vi "MixAndDownsample_5772.vi"(9 "Sine in":fxp<+/-,16,0>[](array[numeric])=[0.0, 0.0, 0.0, 0.0], 10 "Cosine in":fxp<+/-,16,0>[](array[numeric])=[0.0, 0.0, 0.0, 0.0], 11 "Signal Input":i16[](array[numeric])=[0, 0, 0, 0]) -> (0 "data valid":bool, 1 "Q out":fxp<+/-,16,14>, 2 "I out":fxp<+/-,16,14>)   [LabVIEW 2013]
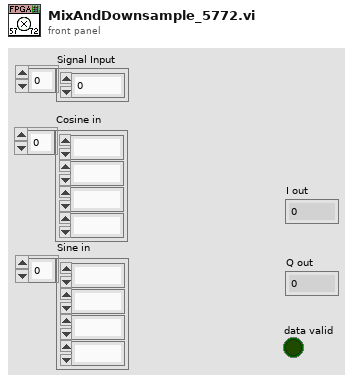
[diagram p1: front panel]
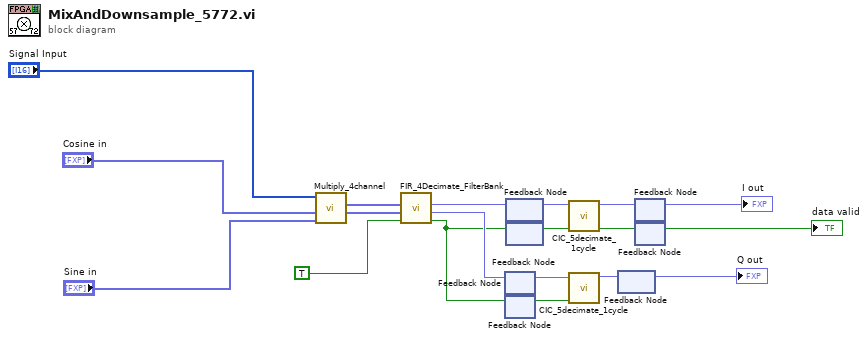
[diagram p0: block diagram]
diagram:
  n1 = call "Multiply_4channel.vi"("DDS Sine"="Sine in", "DDS Cosine"="Cosine in", "Signal Input"="Signal Input") -> ("Q output"=w15:fxp<+/-,16,14>[], "I output"=w16:fxp<+/-,16,14>[])  [unwired: 7 in]
  n2 = call "FIR_4Decimate_FilterBank.vi"("data valid in"=TRUE ("valid in"), "Q in"=w15, "I in"=w16) -> ("data valid out"=w1:bool, "Q out"=w8:fxp<+/-,16,14>, "I out"=w13:fxp<+/-,16,14>)  [unwired: 6 in]
  n3 = feedback #1() -> (w7:fxp<+/-,16,14>)  [unwired: 1 in]
  n4 = feedback-in #1(w8) -> ()
  n5 = feedback #2() -> (w6:bool)  [unwired: 1 in]
  n6 = feedback-in #2(w1) -> ()
  n7 = feedback-in #3(w13) -> ()
  n8 = feedback #3() -> (w12:fxp<+/-,16,14>)  [unwired: 1 in]
  n9 = feedback #4() -> (w11:bool)  [unwired: 1 in]
  n10 = feedback-in #4(w1) -> ()
  n11 = call "CIC_5decimate_1cycle.vi"("valid in"=w11, "Data in"=w12) -> ("valid out"=w3:bool, "Data out"=w5:fxp<+/-,16,14>)  [unwired: 7 in, 1 out]
  n12 = call "CIC_5decimate_1cycle.vi"("valid in"=w6, "Data in"=w7) -> ("Data out"=w10:fxp<+/-,16,14>)  [unwired: 7 in, 2 out]
  n13 = feedback #5() -> (→"Q out":fxp<+/-,16,14>)  [unwired: 1 in]
  n14 = feedback-in #5(w10) -> ()
  n15 = feedback #6() -> (→"I out":fxp<+/-,16,14>)  [unwired: 1 in]
  n16 = feedback-in #6(w5) -> ()
  n17 = feedback #7() -> (→"data valid":bool)  [unwired: 1 in]
  n18 = feedback-in #7(w3) -> ()
